vi "GlobalSetNumberOfDigits_PhysikalInstruments.vi"() -> ()   [LabVIEW 2011]
panel:
  in  "NumberOfDigits Mirror":i32=15 min=1 max=15 step=1
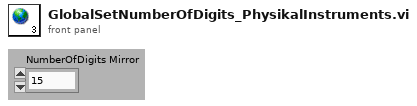
[diagram p1: front panel]
diagram:
